vi "board evaluation.vi"(7 "tic tac toe data in":T1={"state"=enum."start game", "display board"=[], "eval board"=[[0, 0, 0], [0, 0, 0], [0, 0, 0]], "turn"=enum."x turn", "desired move"=[], "game status"=enum."not over"}) -> (8 "tic tac toe data out":T1)   [LabVIEW 2019]
doc: "eval Board determine where move will go and if x or o wins also deterimnes if ongoing, stalemate, and board filled.\n\nJuan Gamez\nP3600\nCsusb Physics"
uses:
  typedefs/tic-tac-toe data.ctl
  typedefs/tic-tac-toe state enum.ctl
  typedefs/turn enum.ctl
  typedefs/game status.ctl
panel:
  out "sum array":i32[](array[numeric])
  out "stalemate":bool
  out "board filled":bool
  out "ongoing":bool
  out "o wins":bool
  out "x wins":bool
  # "row 0"
  # "row 1"
  # "row 2"
  # "column 0"
  # "column 1"
  # "column 2"
  # "diagonal ul"
  # "diagonal ur"
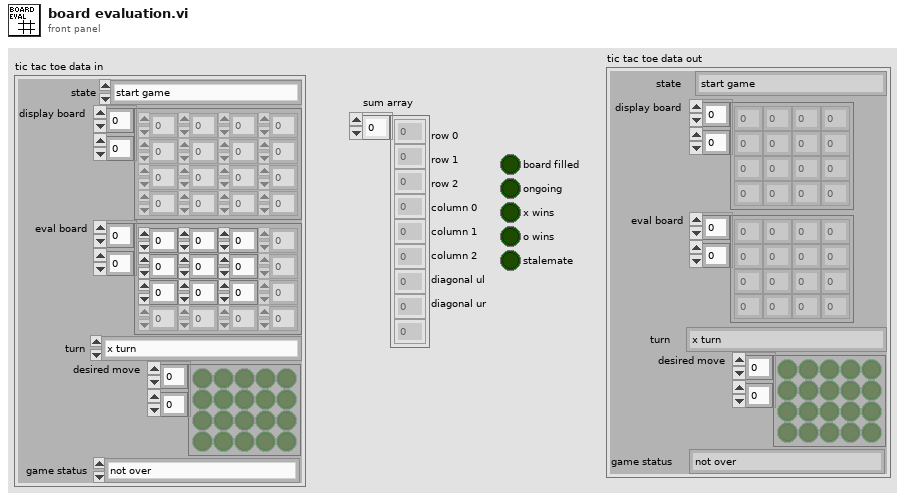
[diagram p1: front panel]
types:
  T1 = typedef "tic-tac-toe data.ctl" = cluster{"state":T2, "display board":u16[][], "eval board":i32[][], "turn":T3, "desired move":bool[][], "game status":T4}
  T2 = typedef "tic-tac-toe state enum.ctl" = enum16{"start game", "clear", "x turn", "o turn", "legal move", "update board", "evaluate board", "turn decide", "game over"}
  T3 = typedef "turn enum.ctl" = enum32{"x turn", "o turn"}
  T4 = typedef "game status.ctl" = enum16{"not over", "over stalemate", "over x wins", "over o wins"}
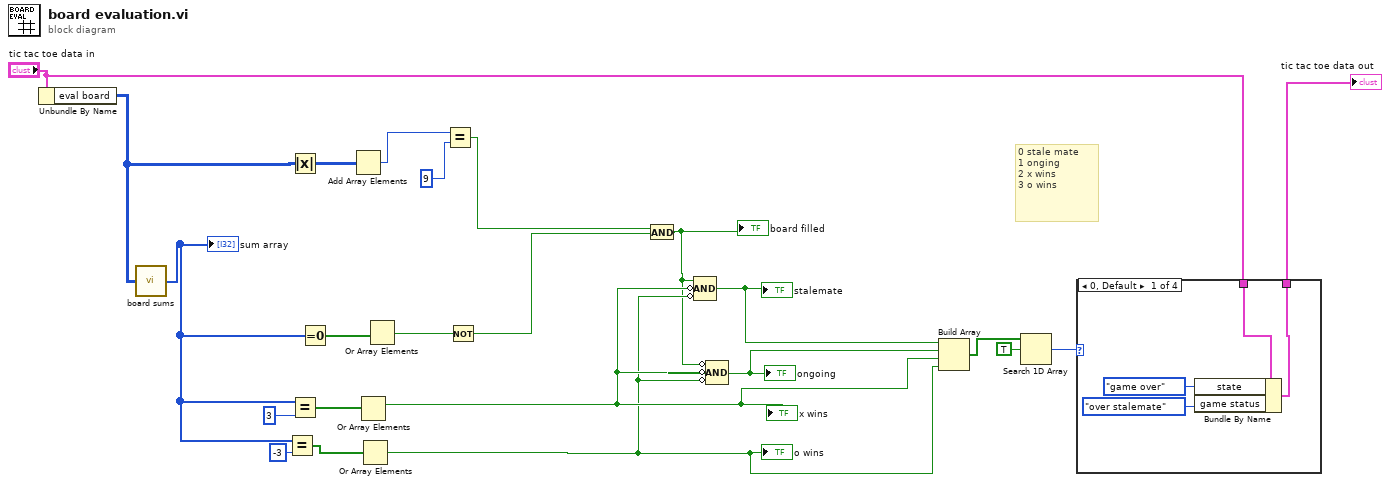
[diagram p0: block diagram]
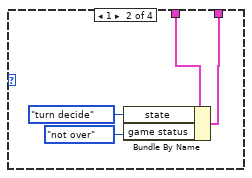
[diagram p2: hidden frame]
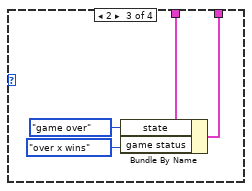
[diagram p3: hidden frame]
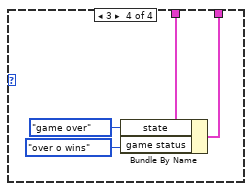
[diagram p4: hidden frame]
diagram:
  # "0 stale mate \n1 onging\n2 x wins \n3 o wins"
  n1 = Unbundle By Name("tic tac toe data in") -> ("eval board"=w1:i32[][])
  n2 = call "board sums.vi"("eval board in"=w1) -> ("sum array"=w2:i32[])  [unwired: 14 in]
  "sum array" <- w2
  n3 = Equal?(x=w2, y=-3) -> (x = y?=w20:bool[])
  n4 = Absolute Value(x=w1) -> (abs(x)=w3:i32[][])
  n5 = Equal?(x=w2, y=3) -> (x = y?=w21:bool[])
  n6 = Equal To 0?(x=w2) -> (x = 0?=w9:bool[])
  n7 = Add Array Elements(numeric array=w3) -> (sum=w6:i32)
  n8 = Or Array Elements(Boolean array=w21) -> (logical OR=w12:bool)
  "x wins" <- w12
  n9 = Or Array Elements(Boolean array=w20) -> (logical OR=w11:bool)
  "o wins" <- w11
  n10 = Or Array Elements(Boolean array=w9) -> (logical OR=w10:bool)
  n11 = Equal?(x=w6, y=9) -> (x = y?=w5:bool)
  n12 = Not(x=w10) -> (.not. x?=w8:bool)
  n13 = And(x=w5, y=w8) -> (x .and. y?=w4:bool)
  "board filled" <- w4
  n14 = Compound Arithmetic op=AND(w4, invert w12, invert w11) -> (w19:bool)
  "stalemate" <- w19
  n15 = Compound Arithmetic op=AND(invert w4, invert w12, invert w11) -> (w18:bool)
  "ongoing" <- w18
  n16 = Build Array(w19, w18, w12, w11) -> (w17:bool[])
  n17 = Search 1D Array(1D array=w17, element=TRUE) -> (index of element=w15:i32)  [unwired: 1 in]
  n18 = case shown="0, Default" w15 {
    tunnel: "tic tac toe data in" -> [w26 w29 w35 w39]
    tunnel: [w25 w28 w34 w38] -> w13
    frame 0, Default {
      n19 = Bundle By Name(cluster=w26, "state"=tic-tac-toe_state_enum."game over", "game status"=game_status."over stalemate") -> (w25:T1)
    }
    frame 1 {
      n20 = Bundle By Name(cluster=w29, "state"=tic-tac-toe_state_enum."turn decide", "game status"=game_status."not over") -> (w28:T1)
    }
    frame 2 {
      n21 = Bundle By Name(cluster=w35, "state"=tic-tac-toe_state_enum."game over", "game status"=game_status."over x wins") -> (w34:T1)
    }
    frame 3 {
      n22 = Bundle By Name(cluster=w39, "state"=tic-tac-toe_state_enum."game over", "game status"=game_status."over o wins") -> (w38:T1)
    }
  }
  "tic tac toe data out" <- w13
